vi "WILT Update Aisle Info.vi"(9 "Aisle 4 Update":T1 {"Night Cycle Count" format="%04d"; "Day Cycle Count" format="%04d"}, 10 "Aisle 4 Location":i32, 11 "GUI Aisle 4. in":T1[](array[typedef]) {"Night Cycle Count" format="%04d"; "Day Cycle Count" format="%04d"}) -> (3 "GUI Aisle 4. out":T1[](array[typedef]) {"Night Cycle Count" format="%04d"; "Day Cycle Count" format="%04d"})   [LabVIEW 2016]
uses:
  Type Definitions/WILT Dryer.ctl
  Type Definitions/WILT Dryer Details.ctl
  Type Definitions/WILT Agilent Channel Definition.ctl
  Type Definitions/WILT DAQ Data.ctl
  <vilib>/Utility/error.llb/whitespace.ctl
panel:
  # "Day"
  # "Night"
  # "Day"
  # "Night"
  # "Day"
  # "Night"
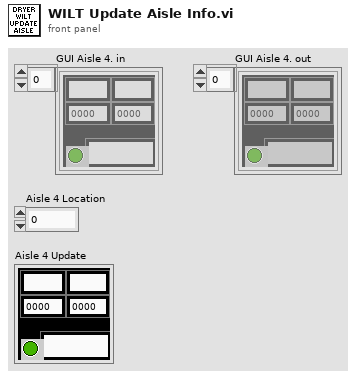
[diagram p1: front panel]
types:
  T1 = typedef "WILT Dryer.ctl" = cluster{"Lab ID":string, "Day Cycle Count":i32, "Station Label":string, "Dryer Details":T2, "Status Color":u32, "Invisible Button":bool, "Night Cycle Count":i32, "Station Index":i32, "Cycle Index":string, "Audit Alert":bool, "Agilent Channel Definition":T3, "DAQ Data":T4}
  T2 = typedef "WILT Dryer Details.ctl" = cluster{"Station":string, "Lab ID":string, "TR Number":string}
  T3 = typedef "WILT Agilent Channel Definition.ctl" = cluster{"Channel":string, "Station":string, "Label":string, "Agilent Station":string, "Data":dbl}
  T4 = typedef "WILT DAQ Data.ctl" = cluster{"L1 Current":dbl, "L2 Current":dbl, "Temperature  Deg F (TC)":dbl, "Volts":dbl, "Volts (208)":dbl, "SW (208)":dbl}
  T5 = typedef "whitespace.ctl" = u16
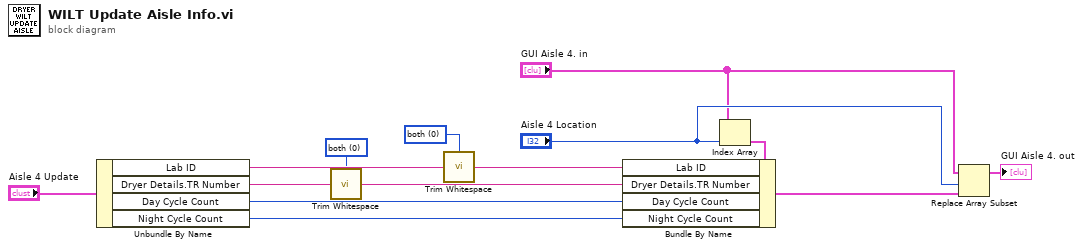
[diagram p0: block diagram]
diagram:
  w1 = T5 0 items=["both", "start of string", "end of string"] ("location (both)")
  w2 = T5 0 items=["both", "start of string", "end of string"] ("location (both)")
  n1 = Unbundle By Name("Aisle 4 Update") -> ("Lab ID"=w6:string, "Dryer Details.TR Number"=w4:string, "Day Cycle Count"=w9:i32, "Night Cycle Count"=w10:i32)
  n2 = call <vilib>:"Trim Whitespace.vi"("string"=w4, "location (both)"=w2) -> ("trimmed string"=w3:string)
  n3 = call <vilib>:"Trim Whitespace.vi"("string"=w6, "location (both)"=w1) -> ("trimmed string"=w5:string)
  n4 = Index Array(array="GUI Aisle 4. in", index="Aisle 4 Location") -> (element=w8:T1)
  n5 = Bundle By Name(cluster=w8, "Lab ID"=w5, "Dryer Details.TR Number"=w3, "Day Cycle Count"=w9, "Night Cycle Count"=w10) -> (w12:T1)
  n6 = Replace Array Subset(array="GUI Aisle 4. in", new element=w12, index="Aisle 4 Location") -> (→"GUI Aisle 4. out":T1[])
